vi "RIMAS Detector SCP File To Server.vi"(8 "Error In":errorcluster, 10 "Detector Computer":T1={"Machine"="192.168.121.11", "Password"="rSL!nux54321", "FITS File Path"="/local/data/fermi-grb1/home/rimas/dev/h2rg/fitdat", "Port"=44444, "Header Path"="/local/data/fermi-grb1/home/rimas/dev/h2rg/header", "Name"=""}, 11 "Local File Path":path=path "C:/Users/ZODI/Documents/LabVIEW Data/FITS Files") -> (0 "Error Out":errorcluster, 3 "cmd line":string)   [LabVIEW 2024]
uses:
  RIMAS Detector Server Config.ctl
panel:
  out "standard error":string
  out "standard output":string
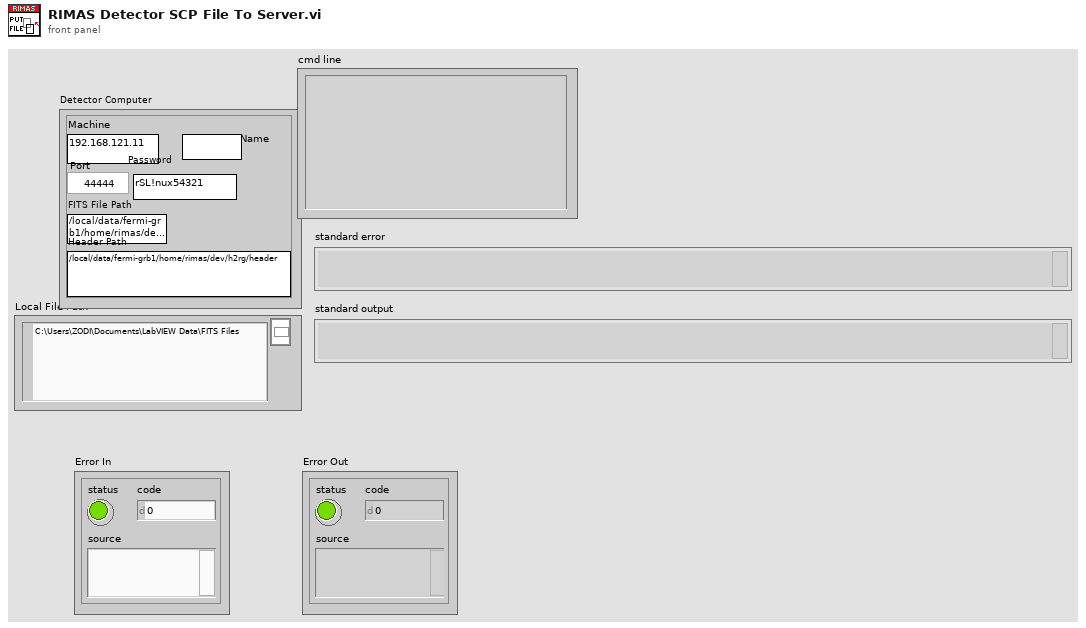
[diagram p1: front panel]
types:
  T1 = typedef "RIMAS Detector Server Config.ctl" = cluster{"Machine":string, "Password":string, "FITS File Path":string, "Port":u16, "Header Path":string, "Name":string}
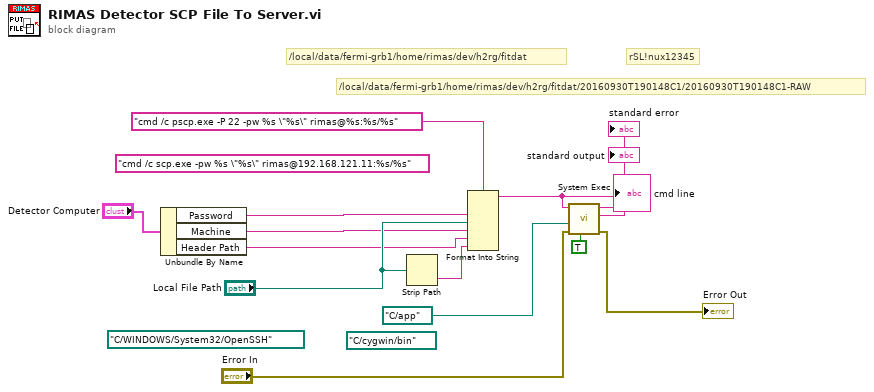
[diagram p0: block diagram]
diagram:
  (unwired) path "C:/WINDOWS/System32/OpenSSH" ("working directory")
  (unwired) path "C:/cygwin/bin" ("working directory")
  (unwired) "cmd /c scp.exe -pw %s \"%s\" rimas@192.168.121.11:%s/%s" ("format string")
  # "/local/data/fermi-grb1/home/rimas/dev/h2rg/fitdat/20160930T190148C1/20160930T190148C1-RAW"
  # "/local/data/fermi-grb1/home/rimas/dev/h2rg/fitdat"
  # "rSL!nux12345"
  n1 = Unbundle By Name("Detector Computer") -> ("Password"=w10:string, "Machine"=w3:string, "Header Path"=w2:string)
  n2 = Strip Path(path="Local File Path") -> (name=w1:string)  [unwired: 1 out]
  n3 = Format Into String(format string="cmd /c pscp.exe -P 22 -pw %s \"%s\" rimas@%s:%s/%s", w10, "Local File Path", w3, w2, w1) -> (resulting string=w14:string)  [unwired: 2 in, 1 out]
  "cmd line" <- w14
  n4 = call <vilib>:"System Exec.vi"("run minimized? (F)"=TRUE, "error in (no error)"="Error In", "working directory"=path "C:/app", "command line"=w14) -> ("error out"=→"Error Out":errorcluster, "standard error"=→"standard error":string, "standard output"=→"standard output":string)  [unwired: 4 in, 1 out]
